vi "RNG ReadState.vi"(8 "error in (no error)":errorcluster, 11 "RNG in":refnum<class "RNG.lvclass">) -> (0 "error out":errorcluster, 2 "State":u64, 3 "RNG out":refnum<class "RNG.lvclass">)   [LabVIEW 2020, in "OpenLvVision_OpenCv.lvlib" / "RNG.lvclass"]
doc: "Read the state from the rng object."
uses:
  RNG.lvclass
  _LvHelpers/EdvrObject/EdvrObject.lvclass
  Dlls/OlvOpenCvWrapper.dll
  C:/Users/lukas/Downloads/OpenLvVision_OpenCv/SourceCode/LabView/OpenLvVision_OpenCv/_LvHelpers/EdvrObject/EdvrObject.lvclass
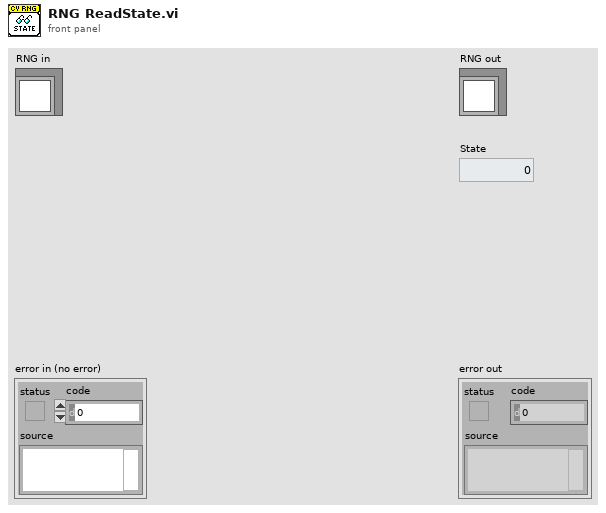
[diagram p1: front panel]
types:
  T1 = typedef "OpenLvVision_OpenCv.lvlib/EdvrObject.lvclass/Edvr.ctl" = refnum<data-value>
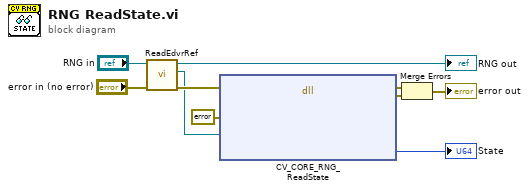
[diagram p0: block diagram]
diagram:
  n1 = call "ReadEdvrRef.vi"("error in (no error)"="error in (no error)", "EdvrObject in"="RNG in") -> ("error out"=w9:errorcluster, "Edvr"=w8:T1, "EdvrObject out"=→"RNG out":refnum<class "RNG.lvclass">)  [unwired: 7 in]
  n2 = dll-call lib="C:/Users/lukas/Downloads/OpenLvVision_OpenCv/SourceCode/LabView/OpenLvVision_OpenCv/Dlls/OlvOpenCvWrapper.dll" fn="CV_CORE_RNG_ReadState"(error in=w9, "Error"=errorcluster {"status"=FALSE, "code"=0, "source"=""} ("error constant"), "edvrRef"=w8) -> (error out=w2:errorcluster, "Error"=w3:errorcluster, "state"=→"State":u64)  [unwired: 5 in, 1 out]
  n3 = Merge Errors(w2, w3) -> (→"error out":errorcluster)
